vi "GetTimeSec.vi"(5 "error in":errorcluster={"status"=FALSE, "code"=1073676294, "source"="VISA Read in CONEC-CC.lvclass:WriteReadSerialPort.vi->CONEC-CC.lvclass:Get Motion Time.vi->Stage Control 01.vi"}) -> (16 "current time":timestamp, 19 "error out":errorcluster={"status"=FALSE, "code"=1073676294, "source"="VISA Read in CONEC-CC.lvclass:WriteReadSerialPort.vi->CONEC-CC.lvclass:Get Motion Time.vi->Stage Control 01.vi"})   [LabVIEW 2017]
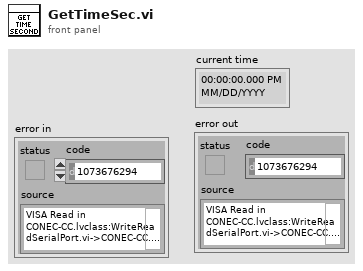
[diagram p1: front panel]
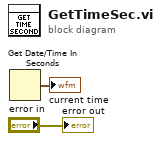
[diagram p0: block diagram]
diagram:
  n1 = Get Date/Time In Seconds() -> (seconds since 1Jan1904=→"current time":timestamp)
  "error out" <- "error in"
